vi "Read.vi"(10 "SMU":dbl, 11 "VISA Refnum in":refnum<visa-resource-name>) -> (2 "Current":dbl, 3 "VISA Refnum out":refnum<visa-resource-name>)   [LabVIEW 2022 SP3]
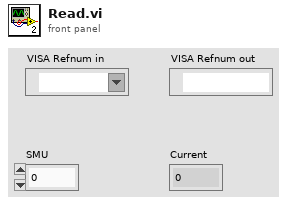
[diagram p1: front panel]
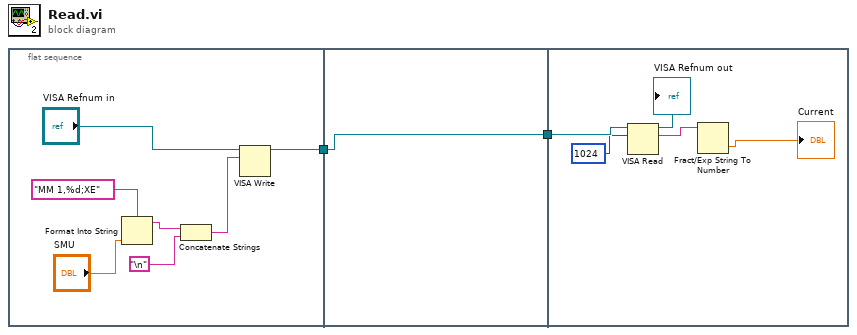
[diagram p0: block diagram]
diagram:
  n1 = flat-sequence {
    tunnel: [w4] -> w2
    tunnel: w2 -> [w10]
    tunnel: [w10] -> w1
    tunnel: w1 -> [w15]
    frame #0 {
      n2 = Format Into String(format string="MM 1,%d;XE", "SMU") -> (resulting string=w7:string)  [unwired: 2 in, 1 out]
      n3 = Concatenate Strings(w7, "\n") -> (w5:string)
      n4 = VISA Write(VISA resource name="VISA Refnum in", write buffer=w5) -> (VISA resource name out=w4:refnum<visa-resource-name>)  [unwired: 1 in, 2 out]
    }
    frame #1 {
    }
    frame #2 {
      n5 = VISA Read(VISA resource name=w15, byte count=u32 1024) -> (VISA resource name out=→"VISA Refnum out":refnum<visa-resource-name>, read buffer=w13:string)  [unwired: 1 in, 2 out]
      n6 = Fract/Exp String To Number(string=w13) -> (number=→"Current":dbl)  [unwired: 3 in, 1 out]
    }
  }
